vi "Klaster_003_PH.vi"() -> ()   [LabVIEW 2021]
panel:
  out "error out":errorcluster={"status"=TRUE, "code"=1430, "source"="Read from Text File in Klaster_003_PH.vi<APPEND>\n"}
  out "source":string="Read from Text File in Klaster_003_PH.vi<APPEND>\n"
  out "code":i32=1430
  out "status":bool=TRUE
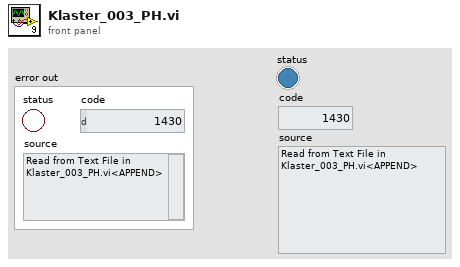
[diagram p1: front panel]
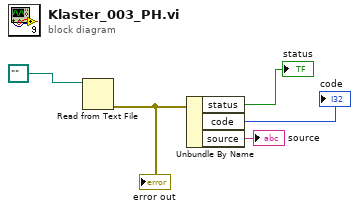
[diagram p0: block diagram]
diagram:
  n1 = Read from Text File(file (use dialog)=path "") -> (error out=w4:errorcluster)  [unwired: 3 in, 3 out]
  "error out" <- w4
  n2 = Unbundle By Name(w4) -> ("status"=→"status":bool, "code"=→"code":i32, "source"=→"source":string)
